vi "Run.vi"(7 "Execution Type":T1, 8 "error in (no error)":errorcluster, 10 "UI Interaction Record (*.ui2r) Filepath":path, 11 "UI_Interaction_Manager in":refnum<class "UI_Interaction_Manager.lvclass">) -> (0 "error out":errorcluster, 3 "UI_Interaction_Manager out":refnum<class "UI_Interaction_Manager.lvclass">)   [LabVIEW 2011, in "UI_Interaction_Manager.lvclass"]
uses:
  UI_Interaction_Manager.lvclass
  TypeDefs/ExecutionType.ctl
  UI_Interaction_Manager.lvclass/UI_Interaction_Manager.ctl
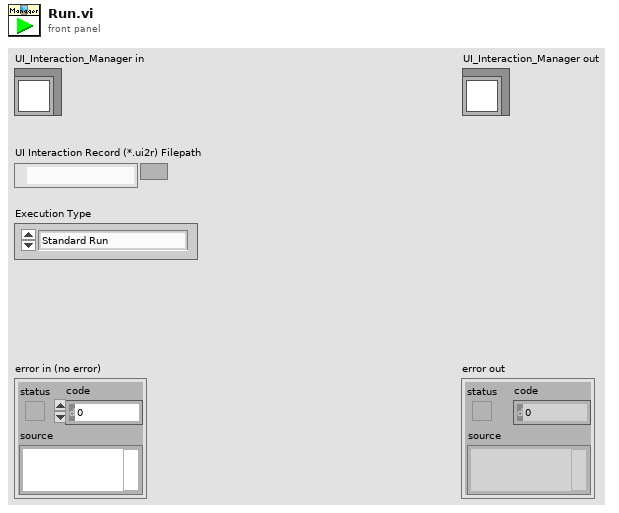
[diagram p1: front panel]
types:
  T1 = typedef "UI_Interaction_Manager.lvclass/ExecutionType.ctl" = enum16{"Standard Run", "Run with Recording", "Auto-Run with Playback"}
  T2 = enum32{"Invalid", "Standard", "Closed", "Hidden", "Minimized", "Maximized"}
  T3 = typedef "UI_Interaction_Manager.lvclass/ControlValueUpdate.ctl" = cluster{"Control Label":string, "Value":variant, "ms":u32}
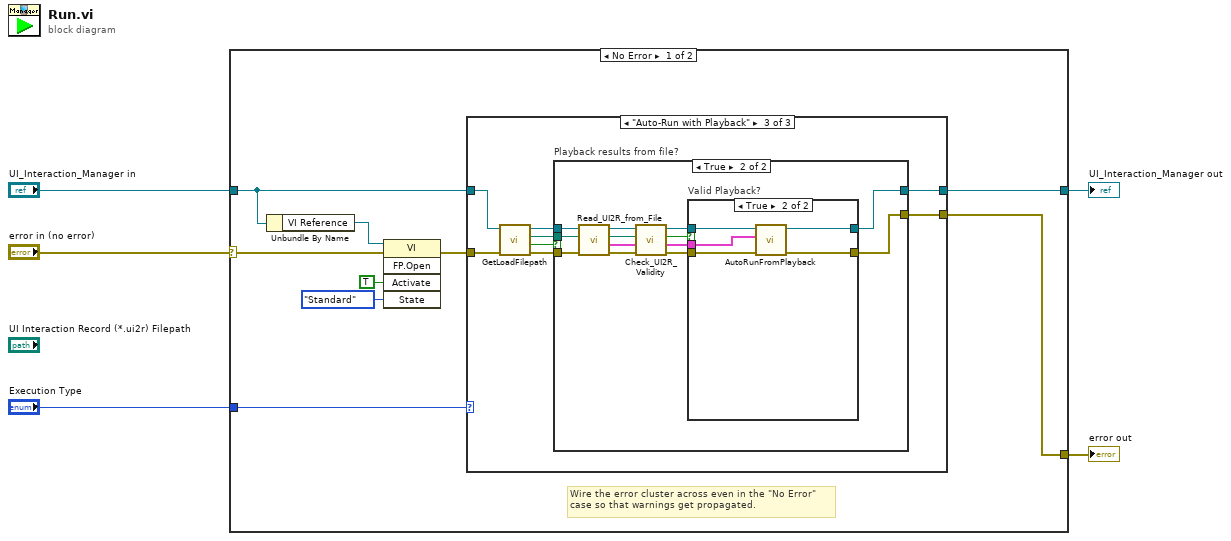
[diagram p0: block diagram]
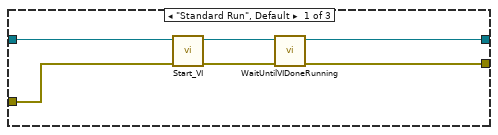
[diagram p2: hidden frame]
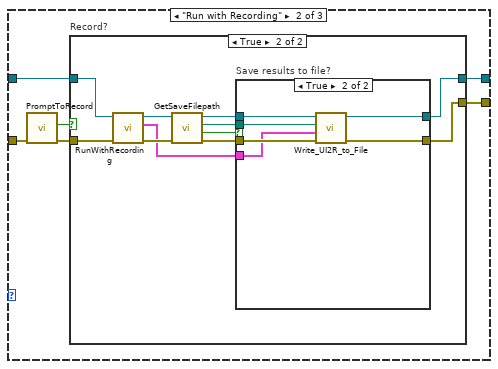
[diagram p3: hidden frame]
diagram:
  n1 = case shown="No Error" "error in (no error)" {
    selector: "error in (no error)" -> [w11 w79]
    tunnel: [w6 w79] -> w4
    tunnel: [w7 w78] -> w2
    tunnel: "UI_Interaction_Manager in" -> [w8 w78]
    tunnel: "Execution Type" -> [w9 _]
    frame No Error {
      # "Wire the error cluster across even in the \"No Error\"\ncase so that warnings get propagated."
      n2 = Unbundle By Name(w8) -> ("VI Reference"=w12:refnum<vi>)
      n3 = invoke class="VI" method="FP.Open"(reference=w12, error in=w11, "Activate"=TRUE ("Activate?"), "State"=T2."Standard") -> (error out=w10:errorcluster)  [unwired: 1 in, 4 out]
      n4 = case shown="\"Auto-Run with Playback\"" w9 {
        tunnel: w10 -> [w19 w26 w55]
        tunnel: w8 -> [w20 w24 w54]
        tunnel: [w16 w22 w49] -> w7
        tunnel: [w15 w21 w48] -> w6
        frame "Standard Run", Default {
          n5 = call "Start_VI.vi"("error in (no error)"=w19, "UI_Interaction_Manager in"=w20) -> ("error out"=w17:errorcluster, "UI_Interaction_Manager out"=w18:refnum<class "UI_Interaction_Manager.lvclass">)  [unwired: 8 in]
          n6 = call "WaitUntilVIDoneRunning.vi"("error in (no error)"=w17, "UI_Interaction_Manager in"=w18) -> ("error out"=w15:errorcluster, "UI_Interaction_Manager out"=w16:refnum<class "UI_Interaction_Manager.lvclass">)  [unwired: 8 in]
        }
        frame "Run with Recording" {
          n7 = call "PromptToRecord.vi"("error in (no error)"=w26) -> ("error out"=w23:errorcluster, "Record?"=w25:bool)  [unwired: 9 in]
          n8 = case "Record?" shown="True" w25 {
            tunnel: w24 -> [w28 w39]
            tunnel: w23 -> [w27 w38]
            tunnel: [w28 w30] -> w22
            tunnel: [w27 w29] -> w21
            frame False {
            }
            frame True {
              n9 = call "RunWithRecording.vi"("error in (no error)"=w38, "UI_Interaction_Manager in"=w39) -> ("error out"=w36:errorcluster, "ControlValueUpdates[]"=w31:T3[], "UI_Interaction_Manager out"=w37:refnum<class "UI_Interaction_Manager.lvclass">)  [unwired: 7 in]
              n10 = call "GetSaveFilepath.vi"("error in (no error)"=w36, "UI_Interaction_Manager in"=w37) -> ("error out"=w34:errorcluster, "OK?"=w35:bool, "Selected Filepath"=w32:path, "UI_Interaction_Manager out"=w33:refnum<class "UI_Interaction_Manager.lvclass">)  [unwired: 6 in]
              n11 = case "Save results to file?" shown="True" w35 {
                tunnel: w34 -> [w40 w47]
                tunnel: w33 -> [w41 w45]
                tunnel: w32 -> [_ w46]
                tunnel: w31 -> [_ w44]
                tunnel: [w41 w43] -> w30
                tunnel: [w40 w42] -> w29
                frame False {
                }
                frame True {
                  n12 = call "Write_UI2R_to_File.vi"("error in (no error)"=w47, "ControlValueUpdates[]"=w44, "UI2R Save Filepath"=w46, "UI_Interaction_Manager in"=w45) -> ("error out"=w42:errorcluster, "UI_Interaction_Manager out"=w43:refnum<class "UI_Interaction_Manager.lvclass">)  [unwired: 6 in]
                }
              }
            }
          }
        }
        frame "Auto-Run with Playback" {
          n13 = call "GetLoadFilepath.vi"("error in (no error)"=w55, "UI_Interaction_Manager in"=w54) -> ("error out"=w50:errorcluster, "Valid?"=w53:bool, "Selected Filepath"=w51:path, "UI_Interaction_Manager out"=w52:refnum<class "UI_Interaction_Manager.lvclass">)  [unwired: 6 in]
          n14 = case "Playback results from file?" shown="True" w53 {
            tunnel: w52 -> [w57 w70]
            tunnel: w51 -> [_ w68]
            tunnel: w50 -> [w56 w69]
            tunnel: [w57 w59] -> w49
            tunnel: [w56 w58] -> w48
            frame False {
            }
            frame True {
              n15 = call "Read_UI2R_from_File.vi"("error in (no error)"=w69, "UI2R Save Filepath"=w68, "UI_Interaction_Manager in"=w70) -> ("error out"=w64:errorcluster, "ControlValueUpdates[]"=w65:T3[], "UI Filepath"=w66:path, "UI_Interaction_Manager out"=w67:refnum<class "UI_Interaction_Manager.lvclass">)  [unwired: 5 in]
              n16 = call "Check_UI2R_Validity.vi"("error in (no error)"=w64, "ControlValueUpdates[] in"=w65, "UI Filepath in"=w66, "UI_Interaction_Manager in"=w67) -> ("error out"=w60:errorcluster, "ControlValueUpdates[] out"=w61:T3[], "Valid?"=w63:bool, "UI_Interaction_Manager out"=w62:refnum<class "UI_Interaction_Manager.lvclass">)  [unwired: 4 in]
              n17 = case "Valid Playback?" shown="True" w63 {
                tunnel: w62 -> [w72 w77]
                tunnel: w61 -> [_ w75]
                tunnel: w60 -> [w71 w76]
                tunnel: [w72 w74] -> w59
                tunnel: [w71 w73] -> w58
                frame False {
                }
                frame True {
                  n18 = call "AutoRunFromPlayback.vi"("error in (no error)"=w76, "ControlValueUpdates[] in"=w75, "UI_Interaction_Manager in"=w77) -> ("error out"=w73:errorcluster, "UI_Interaction_Manager out"=w74:refnum<class "UI_Interaction_Manager.lvclass">)  [unwired: 7 in]
                }
              }
            }
          }
        }
      }
    }
    frame Error {
    }
  }
  "error out" <- w4
  "UI_Interaction_Manager out" <- w2
